vi "Timer With Pause.vi"(7 "Timer Action":T1, 8 "error in (no error)":errorcluster, 10 "Target Time":dbl) -> (0 "error out":errorcluster, 1 "CountDown Time":dbl format="%.2g", 2 "Elapsed Time":dbl format="%.2g", 3 "Done?":bool)   [LabVIEW 2018]
doc: "Use this template to build a VI to use as a subVI."
uses:
  Controls/Timer Actions ENUM_TEST_TDef.ctl
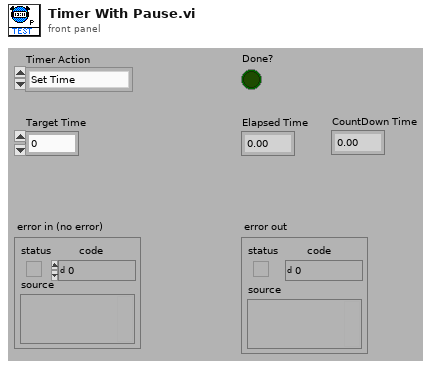
[diagram p1: front panel]
types:
  T1 = typedef "Timer Actions ENUM_TEST_TDef.ctl" = enum16{"Set Time", "Get Time", "Pause Time", "Resume Time"}
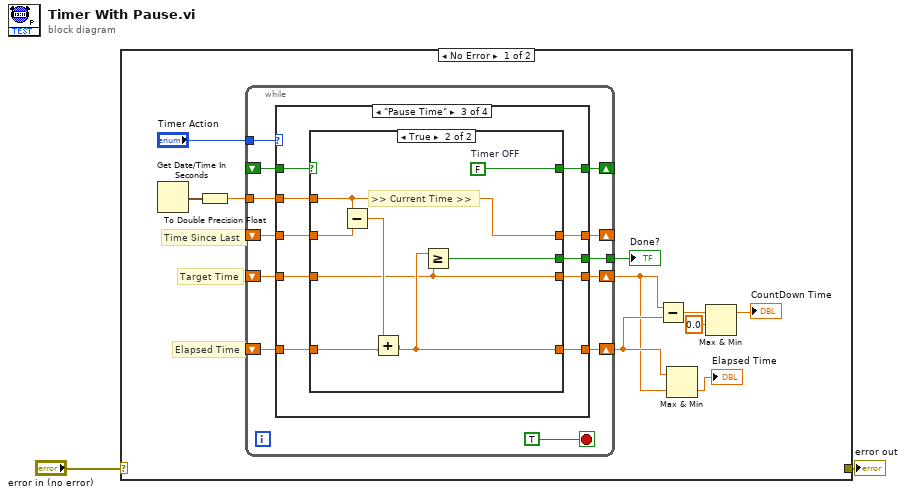
[diagram p0: block diagram]
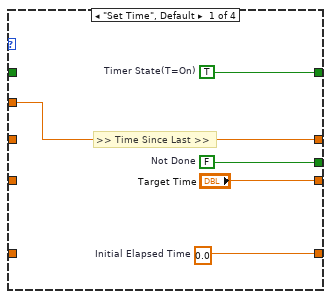
[diagram p2: hidden frame]
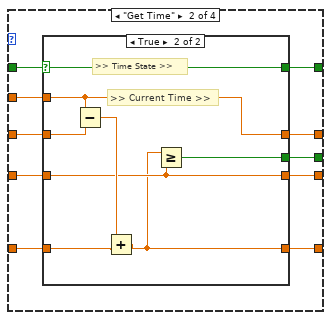
[diagram p3: hidden frame]
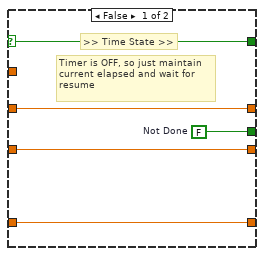
[diagram p4: hidden frame]
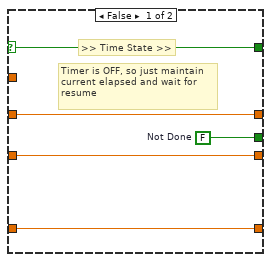
[diagram p5: hidden frame]
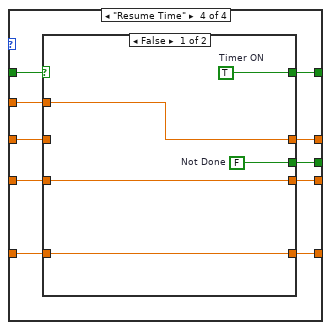
[diagram p6: hidden frame]
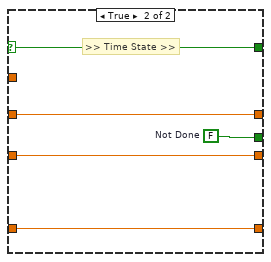
[diagram p7: hidden frame]
diagram:
  n1 = case shown="No Error" "error in (no error)" {
    selector: "error in (no error)" -> [_ w96]
    tunnel: [_ w96] -> w1
    frame No Error {
      # "Elapsed Time"
      # "Target Time"
      # "Time Since Last"
      n2 = Get Date/Time In Seconds() -> (seconds since 1Jan1904=w12:timestamp)
      n3 = To Double Precision Float(number=w12) -> (double precision float=w11:dbl)
      n4 = while {
        tunnel: w11 -> [w18]
        shift-right: [w22] -> w5
        shift-left: _ -> [w21]
        tunnel: "Timer Action" -> [w23]
        shift-right: [w20] -> _
        shift-left: _ -> [w19]
        shift-right: [w17] -> _
        shift-left: _ -> [w15]
        shift-right: [w16] -> w4
        shift-left: _ -> [w14]
        tunnel: [w13] -> w9
        stop <- TRUE stop-if-true
        n5 = case shown="\"Pause Time\"" w23 {
          tunnel: [w29 w36 w60 w83] -> w22
          tunnel: w21 -> [_ w37 w61 w84]
          tunnel: [w28 w32 w57 w80] -> w20
          tunnel: w19 -> [_ w33 w56 w79]
          tunnel: w18 -> [w27 w38 w55 w78]
          tunnel: [w27 w31 w54 w77] -> w17
          tunnel: ["Target Time" w30 w53 w76] -> w16
          tunnel: w15 -> [_ w39 w62 w85]
          tunnel: w14 -> [_ w35 w59 w82]
          tunnel: [w25 w34 w58 w81] -> w13
          frame "Set Time", Default {
            w25 = FALSE  # Not Done
            w28 = TRUE  # Timer State(T=On)
            w29 = 0.0  # Initial Elapsed Time
            # ">> Time Since Last >>"
          }
          frame "Get Time" {
            n6 = case shown="True" w33 {
              selector: w33 -> [w41 w48]
              tunnel: w39 -> [w42 w52]
              tunnel: w38 -> [_ w47]
              tunnel: w37 -> [w44 w51]
              tunnel: [w44 w45] -> w36
              tunnel: w35 -> [w43 w46]
              tunnel: [w40 w49] -> w34
              tunnel: [w41 w48] -> w32
              tunnel: [w42 w47] -> w31
              tunnel: [w43 w46] -> w30
              frame False {
                w40 = FALSE  # Not Done
                # "Timer is OFF, so just maintain\ncurrent elapsed and wait for\nresume"
                # ">> Time State >>"
              }
              frame True {
                # ">> Current Time >>"
                # ">> Time State >>"
                n7 = Subtract(x=w47, y=w52) -> (x-y=w50:dbl)
                n8 = Add(x=w50, y=w51) -> (x+y=w45:dbl)
                n9 = Greater Or Equal?(x=w45, y=w46) -> (x >= y?=w49:bool)
              }
            }
          }
          frame "Pause Time" {
            n10 = case shown="True" w56 {
              selector: w56 -> [w67 _]
              tunnel: w62 -> [w66 w75]
              tunnel: w55 -> [_ w71]
              tunnel: w61 -> [w64 w74]
              tunnel: [w64 w70] -> w60
              tunnel: w59 -> [w65 w69]
              tunnel: [w63 w68] -> w58
              tunnel: [w67 w72] -> w57
              tunnel: [w66 w71] -> w54
              tunnel: [w65 w69] -> w53
              frame False {
                w63 = FALSE  # Not Done
                # "Timer is OFF, so just maintain\ncurrent elapsed and wait for\nresume"
                # ">> Time State >>"
              }
              frame True {
                w72 = FALSE  # Timer OFF
                # ">> Current Time >>"
                n11 = Subtract(x=w71, y=w75) -> (x-y=w73:dbl)
                n12 = Add(x=w73, y=w74) -> (x+y=w70:dbl)
                n13 = Greater Or Equal?(x=w70, y=w69) -> (x >= y?=w68:bool)
              }
            }
          }
          frame "Resume Time" {
            n14 = case shown="False" w79 {
              selector: w79 -> [_ w94]
              tunnel: w85 -> [_ w91]
              tunnel: w78 -> [w86 _]
              tunnel: w84 -> [w89 w93]
              tunnel: [w89 w93] -> w83
              tunnel: w82 -> [w90 w95]
              tunnel: [w88 w92] -> w81
              tunnel: [w87 w94] -> w80
              tunnel: [w86 w91] -> w77
              tunnel: [w90 w95] -> w76
              frame False {
                w87 = TRUE  # Timer ON
                w88 = FALSE  # Not Done
              }
              frame True {
                w92 = FALSE  # Not Done
                # ">> Time State >>"
              }
            }
          }
        }
      }
      "Done?" <- w9
      n15 = Subtract(x=w4, y=w5) -> (x-y=w8:dbl)
      n16 = Max & Min(x=w5, y=w4) -> (min(x,y)=→"Elapsed Time":dbl)  [unwired: 1 out]
      n17 = Max & Min(x=w8, y=0.0) -> (max(x,y)=→"CountDown Time":dbl)  [unwired: 1 out]
    }
    frame Error {
    }
  }
  "error out" <- w1
